vi "Get String (inlined).vi"(8 "error in (no error)":errorcluster, 10 "Offset":i32, 11 "JSON":string) -> (0 "error out":errorcluster, 1 "String":string, 2 "Offset past match":i32)   [LabVIEW 2013, in "JSONtext.lvlib"]
uses:
  JSONtext.lvlib
  support/Unescape JSON string.vi
  support/JSONtext support.lvlib
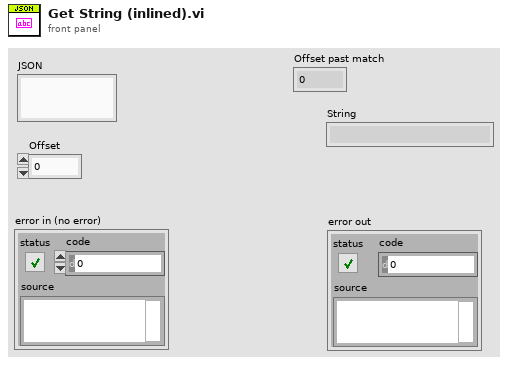
[diagram p1: front panel]
types:
  T1 = typedef "JSONtext.lvlib/Parsing State.ctl" = enum16{"Parser Error", "Object", "Array", "String", "Number/Other", "Leading Whitespace", "Object end", "Array end", "Value end"}
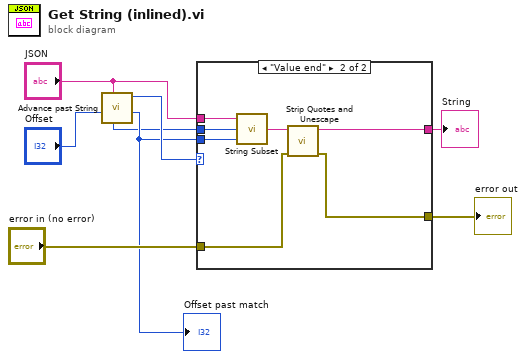
[diagram p0: block diagram]
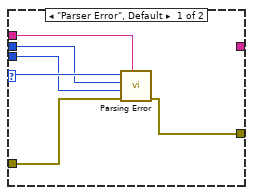
[diagram p2: hidden frame]
diagram:
  n1 = call "Advance past String.vi"("JSON"="JSON", "Offset"="Offset") -> ("Offset past match"=w2:i32, "State"=w6:T1, "Value start out"=w1:i32)  [unwired: 7 in]
  "Offset past match" <- w2
  n2 = case shown="\"Value end\"" w6 {
    selector: w6 -> [w12 _]
    tunnel: "JSON" -> [w9 w20]
    tunnel: [w14 w18] -> w5
    tunnel: "error in (no error)" -> [w13 w19]
    tunnel: [_ w17] -> w3
    tunnel: w1 -> [w11 w16]
    tunnel: w2 -> [w10 w15]
    frame "Parser Error", Default {
      n3 = call "Parsing Error.vi"("JSON"=w9, "error in (no error)"=w13, "Offset past match"=w10, "Value start"=w11, "State"=w12) -> ("error out"=w14:errorcluster)  [unwired: 6 in]
    }
    frame "Value end" {
      n4 = call "String Subset.vi"("Offset past End"=w15, "Start offset"=w16, "JSON"=w20) -> ("substring"=w21:string)  [unwired: 2 in]
      n5 = call "Strip Quotes and Unescape.vi"("error in (no error)"=w19, "String"=w21) -> ("error out"=w18:errorcluster, "result string"=w17:string)  [unwired: 8 in]
    }
  }
  "error out" <- w5
  "String" <- w3
